vi "CMN_GetUTTime.vi"() -> (1 "str time":string, 2 "date time rec":T1)   [LabVIEW 2016]
uses:
  private/c/lib/libcommon.so
panel:
  in  "second":dbl
  in  "minute":i32
  in  "hour":i32
  in  "day":i32
  in  "month":i32
  in  "year":i32
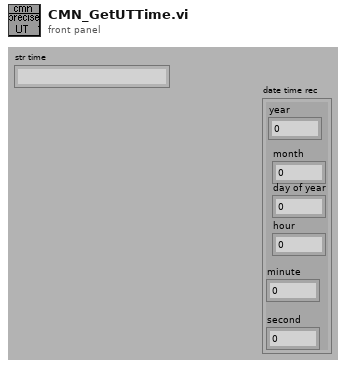
[diagram p1: front panel]
types:
  T1 = cluster{"year":i32, "month ":i32, "day of year":i32, "hour":i32, "minute":i32, "second":dbl}
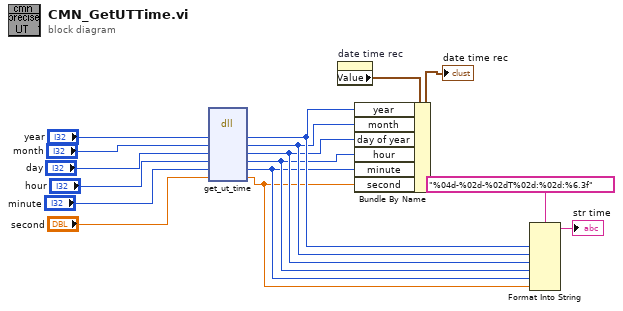
[diagram p0: block diagram]
diagram:
  n1 = dll-call lib="home/simager/panview/PAN/Modules/Common/private/c/lib/libcommon.so" fn="get_ut_time"("year"="year", "month"="month", "day"="day", "hour"="hour", "minute"="minute", "second"="second") -> ("year"=w7:i32, "month"=w6:i32, "day"=w5:i32, "hour"=w4:i32, "minute"=w3:i32, "second"=w2:dbl)  [unwired: 3 in, 3 out]
  n2 = property on="date time rec" class="Clust (strict)"() -> ("Value"=w10:T1)  [unwired: 2 in, 2 out]
  n3 = Bundle By Name(cluster=w10, "year"=w7, "month"=w6, "day of year"=w5, "hour"=w4, "minute"=w3, "second"=w2) -> (→"date time rec":T1)
  n4 = Format Into String(format string="%04d-%02d-%02dT%02d:%02d:%6.3f", w7, w6, w5, w4, w3, w2) -> (resulting string=→"str time":string)  [unwired: 2 in, 1 out]
